vi "NI_PID_demo.vi"(8 "Initialize":bool, 11 "dt (s) in":dbl) -> (3 "dt (s) out":dbl)   [LabVIEW 2010]
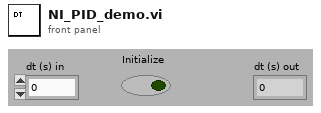
[diagram p1: front panel]
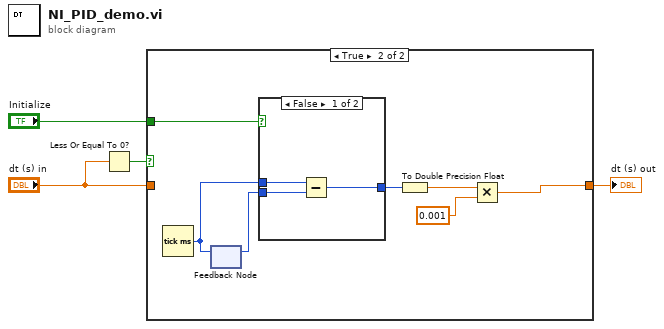
[diagram p0: block diagram]
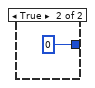
[diagram p3: hidden frame]
diagram:
  n1 = Less Or Equal To 0?(x="dt (s) in") -> (x <= 0?=w2:bool)
  n2 = case shown="True" w2 {
    tunnel: "Initialize" -> [_ w12]
    tunnel: [w5 w6] -> w3
    tunnel: "dt (s) in" -> [w5 _]
    frame False {
    }
    frame True {
      n3 = Tick Count (ms)() -> (millisecond timer value=w11:u32)
      n4 = feedback-in #1(w11) -> ()
      n5 = feedback #1() -> (w10:u32)  [unwired: 1 in]
      n6 = case shown="False" w12 {
        tunnel: w11 -> [w15 _]
        tunnel: w10 -> [w14 _]
        tunnel: [w13 u32 0] -> w9
        frame False {
          n7 = Subtract(x=w15, y=w14) -> (x-y=w13:u32)
        }
        frame True {
        }
      }
      n8 = To Double Precision Float(number=w9) -> (double precision float=w8:dbl)
      n9 = Multiply(x=w8, y=0.001) -> (x*y=w6:dbl)
    }
  }
  "dt (s) out" <- w3
